vi "SVPWMalphabetaFXP.vi"(0 "alpha":fxp<+/-,32,4> caption="voltage alpha", 1 "SVPWMparams":T1={"max"=0.999969482421875, "Period"=0, "Deadtime"=1}, 5 "beta":fxp<+/-,32,4> caption="voltage beta", 9 "input valid":bool=TRUE, 12 "enable":bool=TRUE) -> (4 "SwitchPositions":T2, 14 "Sector":u8, 15 "ready for input":bool)   [LabVIEW 2015, in "SVPWM.lvlib"]
uses:
  SVPWM.lvlib
  SwitchPositions.ctl
  SVPWM_FXP.ctl
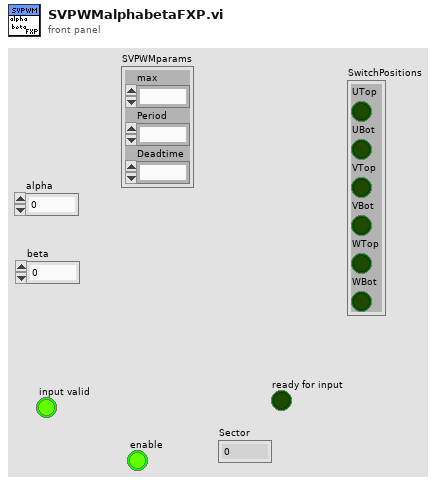
[diagram p1: front panel]
types:
  T1 = typedef "SVPWM.lvlib/SVPWM_FXP.ctl" = cluster{"max":fxp<+/-,32,4>, "Period":u32, "Deadtime":u8}
  T2 = typedef "SVPWM.lvlib/SwitchPositions.ctl" = cluster{"UTop":bool, "UBot":bool, "VTop":bool, "VBot":bool, "WTop":bool, "WBot":bool}
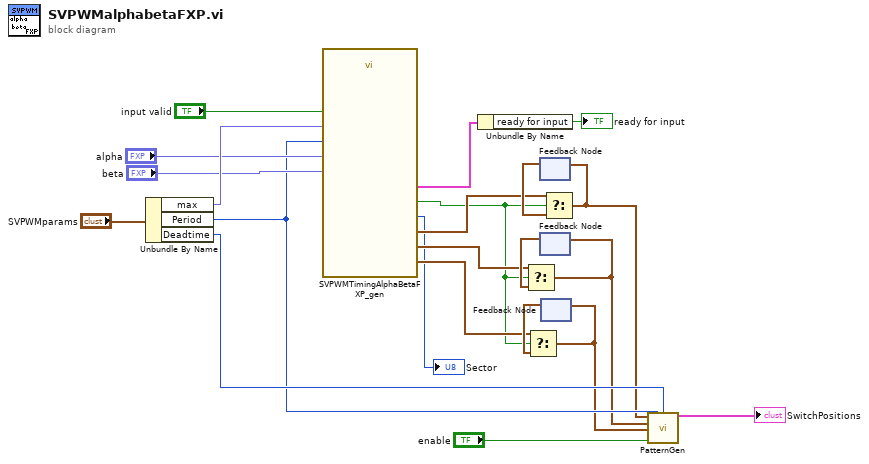
[diagram p0: block diagram]
diagram:
  n1 = Unbundle By Name("SVPWMparams") -> ("max"=w8:fxp<+/-,32,4>, "Period"=w5:u32, "Deadtime"=w15:u8)
  n2 = call "SVPWMTimingAlphaBetaFXP_gen.vi"("beta"="beta", "Period"=w5, "max"=w8, "input valid"="input valid", "alpha"="alpha") -> ("Sector"=→"Sector":u8, "W_timing"=w10:cluster{"ON":u32, "OFF":u32}, "V_Timing"=w11:cluster{"ON":u32, "OFF":u32}, "output valid"=w9:bool, "feedback signals"=w13:cluster{"ready for input":bool}, "U_Timing"=w12:cluster{"ON":u32, "OFF":u32})  [unwired: 5 in]
  n3 = Unbundle By Name(w13) -> ("ready for input"=→"ready for input":bool)
  n4 = feedback #1() -> (w22:cluster{"ON":u32, "OFF":u32})  [unwired: 1 in]
  n5 = feedback #2() -> (w21:cluster{"ON":u32, "OFF":u32})  [unwired: 1 in]
  n6 = Select(t=w11, s=w9, f=w21) -> (s? t:f=w2:cluster{"ON":u32, "OFF":u32})
  n7 = feedback-in #2(w2) -> ()
  n8 = feedback #3() -> (w20:cluster{"ON":u32, "OFF":u32})  [unwired: 1 in]
  n9 = Select(t=w10, s=w9, f=w20) -> (s? t:f=w1:cluster{"ON":u32, "OFF":u32})
  n10 = feedback-in #3(w1) -> ()
  n11 = Select(t=w12, s=w9, f=w22) -> (s? t:f=w3:cluster{"ON":u32, "OFF":u32})
  n12 = feedback-in #1(w3) -> ()
  n13 = call "PatternGen.vi"("U_timing"=w3, "Period"=w5, "Deadtime"=w15, "V_timing"=w2, "W_timing"=w1, "enable"="enable") -> ("SwitchPositions"=→"SwitchPositions":T2)  [unwired: 9 in]
